vi "Read Waveform.vi"(8 "error in":errorcluster, 9 "Transfer Type":i32(ring) items=["s8", "s16", "s32", "f32", "f64"], 10 "Source":i32(ring) items=["Input Channel 1", "Input Channel 2", "Input Channel 3", "Input Channel 4", "Calc Channel 1", "Calc Channel 2", "Calc Channel 3", "Calc Channel 4", "Ref Channel 1", "Ref Channel 2", "Ref Channel 3", "Ref Channel 4"], 11 "Instrument Handle In":i32) -> (0 "error out":errorcluster, 1 "Time":dbl[](array[numeric]), 2 "Waveform":dbl[](array[numeric]), 3 "Instrument Handle Out":i32)   [LabVIEW 8.6, in "ZTScopeM.lvlib"]
doc: "Read the waveform in the source channel."
uses:
  ZTScopeM.lvlib
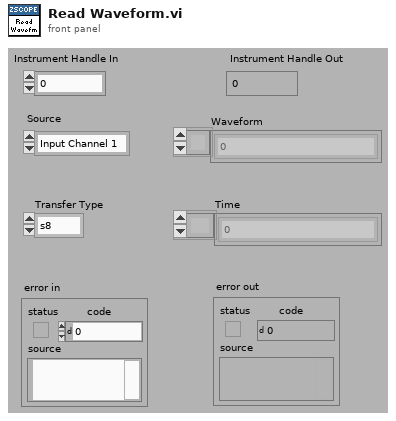
[diagram p1: front panel]
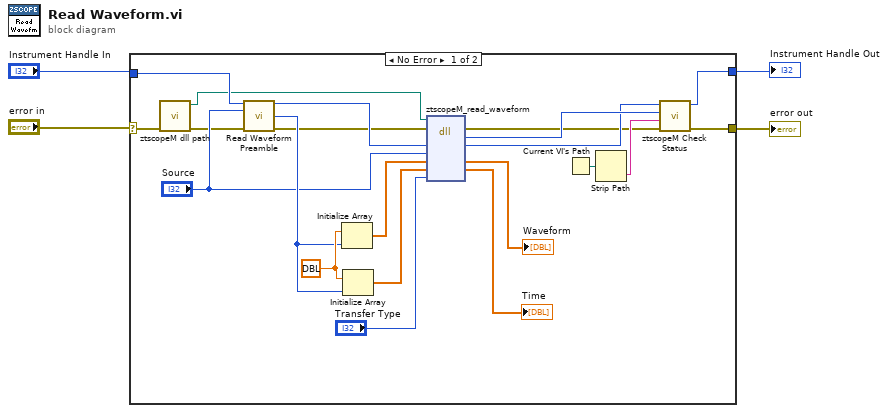
[diagram p0: block diagram]
diagram:
  n1 = case shown="No Error" "error in" {
    selector: "error in" -> [w8 w27]
    tunnel: [w10 w27] -> w1
    tunnel: "Instrument Handle In" -> [w19 w26]
    tunnel: [w11 w26] -> w3
    frame #0 {
      w20 = dbl ?
      n2 = call "ztscopeM dll path.vi"("error in (no error)"=w8) -> ("error out"=w9:errorcluster, "<instrument>.dll path"=w7:path)  [unwired: 9 in]
      n3 = call "Read Waveform Preamble.vi"("Instrument Handle In"=w19, "Source"="Source", "error in"=w9) -> ("Instrument Handle Out"=w18:i32, "Points"=w17:u32, "error out"=w6:errorcluster)  [unwired: 4 in, 6 out]
      n4 = Initialize Array(w20, w17) -> (w22:dbl[])
      n5 = Initialize Array(w20, w17) -> (w21:dbl[])
      n6 = dll-call lib="C:/Program Files (x86)/National Instruments/LabVIEW 2013/instr.lib/ztscopem/ztscopeM.dll" fn="ztscopeM_read_waveform"(path in=w7, error in=w6, "instrumentHandle"=w18, "source"="Source", "Waveform"=w22, "time"=w21, "transferType"="Transfer Type") -> (error out=w5:errorcluster, w13:i32, "instrumentHandle"=w12:i32, "Waveform"=→"Waveform":dbl[], "time"=→"Time":dbl[])  [unwired: 3 in, 1 out]
      n7 = Current VI's Path() -> (path=w15:path)
      n8 = Strip Path(path=w15) -> (name=w14:string)  [unwired: 1 out]
      n9 = call "ztscopeM Check Status.vi"("error in"=w5, "name of VI"=w14, "status (return code)"=w13, "instrument handle in"=w12) -> ("error out"=w10:errorcluster, "instrument handle out"=w11:i32)  [unwired: 2 in]
    }
    frame #1 {
    }
  }
  "Instrument Handle Out" <- w3
  "error out" <- w1
